vi "Verify.vi"   [LabVIEW 2021]
uses:
  RSA/RSA.lvclass
  MD5/MD5.lvclass
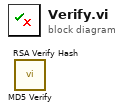
[diagram p0: block diagram]
diagram:
  n1 = call "MD5 Verify.vi"() -> ()  [unwired: 10 in, 2 out]
  n2 = call "RSA Verify Hash.vi"() -> ()  [unwired: 9 in, 3 out]
